vi "Gear Controller.vi"(8 "error in":errorcluster) -> ()   [LabVIEW 2015]
doc: "This VI executes continuously carrying out the current operation and responding to updates or new operations. It will often contain the timing or control code that is difficult to place directly in TeleOp. This VI generally opens all sensors and motors and isolates the rest of the robot code from knowing how the operations are carried out."
uses:
  Gear.ctl
  <vilib>/Rock Robotics/WPI/Solenoid/WPI_SolenoidValue.ctl
  Gear Setpoints.ctl
  Gear Operations.ctl
  <vilib>/Rock Robotics/WPI/Solenoid/WPI_SolenoidChannel.ctl
  Framework/Robot Global Data.vi
  <vilib>/Rock Robotics/WPI/Solenoid/WPI_SolenoidOpenSingle.vi
  <vilib>/Rock Robotics/WPI/Solenoid/WPI_SolenoidSetEnum.vi
panel:
  out "error IO":errorcluster
  in  "Apply Change":bool
  in  "Solenoid 6 (PTO de-active)":T1
  in  "Solenoid 5 (PTO Active)":T1
  in  "Solenoid 4 (Holdball)":T1
  in  "Solenoid 3 (Shootball)":T1
  in  "Solenoid 2 (Gearbox High)":T1
  in  "Solenoid 1 (Gearbox Low)":T1
  out "Gear":T2
  out "Current\nCmd":string
  # "Tip: It may be helpful to observe inputs and sensor values.\nYou may also want to display tuning or debugging controls."
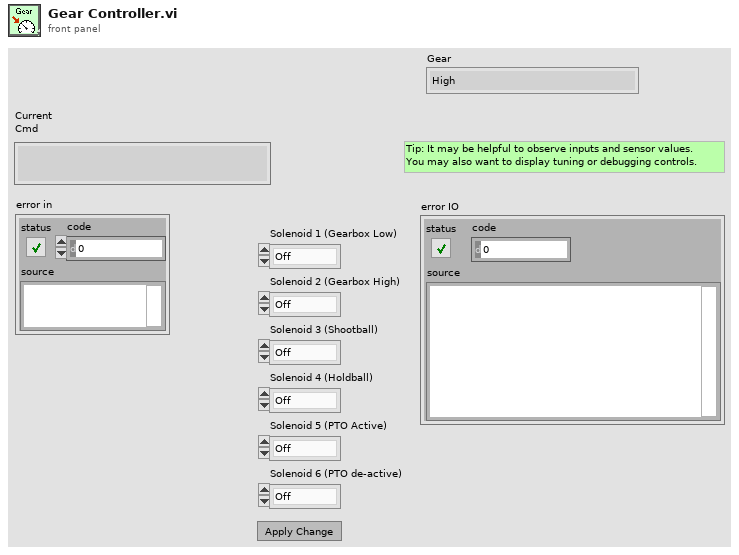
[diagram p1: front panel]
types:
  T1 = typedef "WPI_SolenoidValue.ctl" = enum16{"Off", "On", "Forward", "Reverse"}
  T2 = typedef "Gear.ctl" = enum16{"High", "Low"}
  T3 = typedef "Robot Type Def.ctl" = enum16{"Disabled", "Ghost", "Casper", "Lofty", "Board"}
  T4 = typedef "WPI_SolenoidChannel.ctl" = enum8{"Solenoid 0", "Solenoid 1", "Solenoid 2", "Solenoid 3", "Solenoid 4", "Solenoid 5", "Solenoid 6", "Solenoid 7", "Invalid"}
  T5 = typedef "Gear Setpoints.ctl" = cluster{"Operation":T6, "Setpoint":dbl, "Duration":dbl, "Gear":T2}
  T6 = typedef "Gear Operations.ctl" = enum16{"Reserve", "Read Current", "Immediate", "Change Gear"}
  T7 = typedef "WPI_CompressorDevRef.ctl" = cluster{"DevStatus":errorcluster, "Pneumatics Control Module":u8}
  T8 = typedef "WPI_SolenoidDevRef.ctl" = cluster{"DevStatus":errorcluster, "Pneumatics Control Module":u8, "Forward Solenoid Channel":T4, "Reverse Solenoid Channel":T4}
  T9 = typedef "Command Status Info.ctl" = cluster{"Name":string, "Status":T10, "notifier out":T11}
  T10 = typedef "Completion Status.ctl" = enum16{"Successful", "Aborted", "Incomplete"}
  T11 = typedef "Completion Notifier.ctl" = refnum<notifier>
  T12 = cluster{"Default Command":T5, "Command Timing":cluster{"Start Time (ms)":u32, "Iterations":i32}, "Command Arguments":cluster{"Command Info":T9, "Description":string, "Default Command":T5, "notifier out":refnum<notifier>, "Subsystem Name":string}}
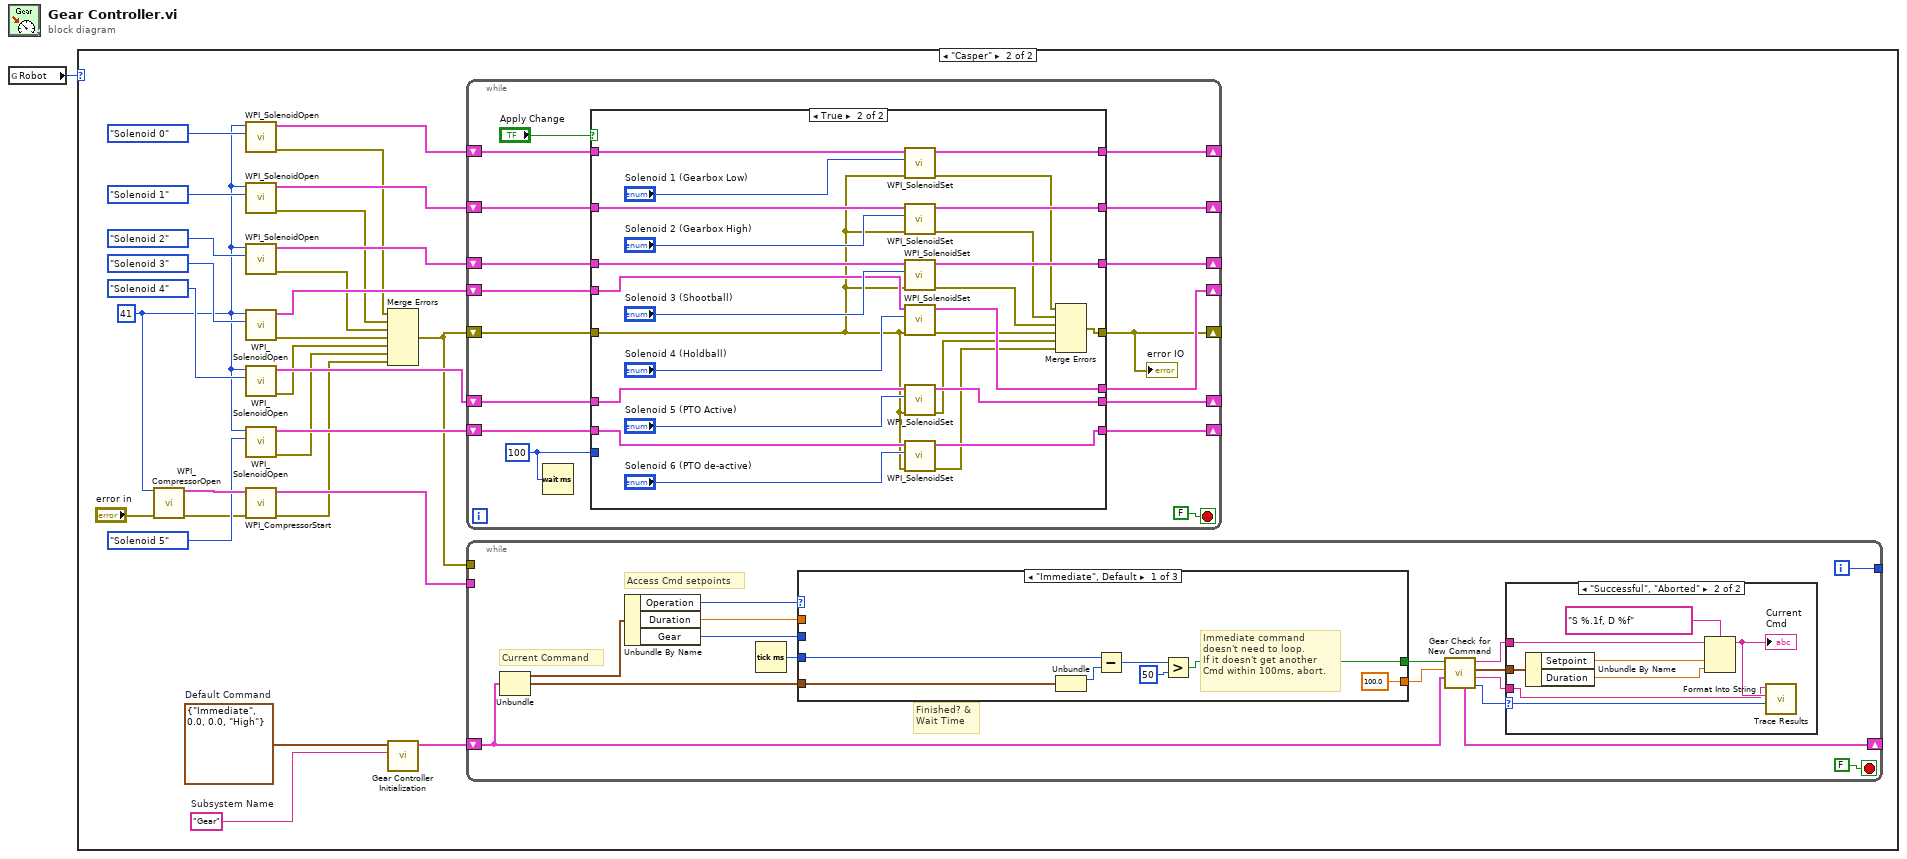
[diagram p0: block diagram]
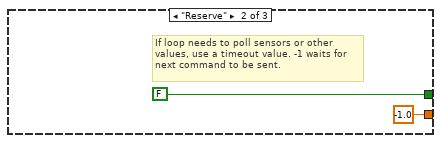
[diagram p5: hidden frame]
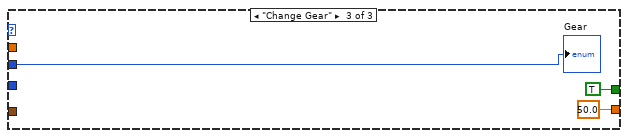
[diagram p6: hidden frame]
diagram:
  n1 = global read "Robot Global Data.vi" "Robot"() -> (w1:T3)
  n2 = case shown="\"Casper\"" w1 {
    frame "Disabled", Default {
    }
    frame "Casper" {
      w17 = u8 41 ("Pneumatics Control Module (0)")
      w27 = T5 {"Operation"=enum."Immediate", "Setpoint"=0.0, "Duration"=0.0, "Gear"=enum."High"}  # Default Command
      w28 = "Gear"  # Subsystem Name
      n3 = call <vilib>:"WPI_CompressorOpen.vi"("Pneumatics Control Module (0)"=w17, "error in (no error)"="error in") -> ("CompressorDevRef"=w26:T7, "error out"=w9:errorcluster)  [unwired: 12 in]
      n4 = call-poly <vilib>:"WPI_SolenoidOpen.vi"("Solenoid Channel"=WPI_SolenoidChannel."Solenoid 0", "Pneumatics Control Module (0)"=w17) -> ("error out"=w2:errorcluster, "SolenoidDevRef"=w23:T8)  [unwired: 8 in]
      n5 = call-poly <vilib>:"WPI_SolenoidOpen.vi"("Solenoid Channel"=WPI_SolenoidChannel."Solenoid 1", "Pneumatics Control Module (0)"=w17) -> ("error out"=w8:errorcluster, "SolenoidDevRef"=w12:T8)  [unwired: 8 in]
      n6 = call-poly <vilib>:"WPI_SolenoidOpen.vi"("Solenoid Channel"=WPI_SolenoidChannel."Solenoid 2", "Pneumatics Control Module (0)"=w17) -> ("error out"=w7:errorcluster, "SolenoidDevRef"=w13:T8)  [unwired: 8 in]
      n7 = call-poly <vilib>:"WPI_SolenoidOpen.vi"("Solenoid Channel"=WPI_SolenoidChannel."Solenoid 3", "Pneumatics Control Module (0)"=w17) -> ("error out"=w6:errorcluster, "SolenoidDevRef"=w14:T8)  [unwired: 8 in]
      n8 = call-poly <vilib>:"WPI_SolenoidOpen.vi"("Solenoid Channel"=WPI_SolenoidChannel."Solenoid 4", "Pneumatics Control Module (0)"=w17) -> ("error out"=w5:errorcluster, "SolenoidDevRef"=w15:T8)  [unwired: 8 in]
      n9 = call-poly <vilib>:"WPI_SolenoidOpen.vi"("Solenoid Channel"=WPI_SolenoidChannel."Solenoid 5", "Pneumatics Control Module (0)"=w17) -> ("error out"=w4:errorcluster, "SolenoidDevRef"=w16:T8)  [unwired: 8 in]
      n10 = call <vilib>:"WPI_CompressorStart.vi"("error in (no error)"=w9, "CompressorDevRef"=w26) -> ("error out"=w3:errorcluster, "CompressorDevRef"=w25:T7)  [unwired: 8 in]
      n11 = Merge Errors(w2, w8, w7, w6, w5, w4, w3) -> (w11:errorcluster)
      n12 = call "Gear Controller Initialization.vi"("Subsystem Name"=w28, "Default Command"=w27) -> ("Command Info"=w29:T12)  [unwired: 9 in]
      n13 = while {
        shift-right: [w45] -> _
        shift-left: w23 -> [w46]
        shift-right: [w39] -> _
        shift-left: w16 -> [w40]
        shift-right: [w38] -> _
        shift-left: w15 -> [w41]
        shift-right: [w37] -> _
        shift-left: w14 -> [w42]
        shift-right: [w36] -> _
        shift-left: w13 -> [w43]
        shift-right: [w35] -> _
        shift-left: w12 -> [w44]
        shift-right: [w32] -> _
        shift-left: w11 -> [w31]
        stop <- FALSE stop-if-true
        w30 = u32 100 ("milliseconds to wait")
        n14 = Wait (ms)(milliseconds to wait=w30) -> ()  [unwired: 1 out]
        n15 = case shown="True" "Apply Change" {
          tunnel: w46 -> [w49 w79]
          tunnel: [w49 w78] -> w45
          tunnel: w44 -> [w50 w75]
          tunnel: w43 -> [w51 w74]
          tunnel: w42 -> [w52 w72]
          tunnel: w41 -> [w53 w69]
          tunnel: w40 -> [w48 w68]
          tunnel: [w48 w66] -> w39
          tunnel: [w53 w65] -> w38
          tunnel: [w52 w64] -> w37
          tunnel: [w51 w63] -> w36
          tunnel: [w50 w62] -> w35
          tunnel: w30 -> [_ _]
          tunnel: [w47 w61] -> w32
          tunnel: w31 -> [w47 w54]
          frame False {
          }
          frame True {
            n16 = call-poly <vilib>:"WPI_SolenoidSet.vi"("error in (no error)"=w54, "Value"="Solenoid 1 (Gearbox Low)", "SolenoidDevRef"=w79) -> ("error out"=w60:errorcluster, "SolenoidDevRef"=w78:T8)  [unwired: 7 in]
            n17 = call-poly <vilib>:"WPI_SolenoidSet.vi"("error in (no error)"=w54, "Value"="Solenoid 2 (Gearbox High)", "SolenoidDevRef"=w75) -> ("error out"=w59:errorcluster, "SolenoidDevRef"=w62:T8)  [unwired: 7 in]
            n18 = call-poly <vilib>:"WPI_SolenoidSet.vi"("error in (no error)"=w54, "Value"="Solenoid 3 (Shootball)", "SolenoidDevRef"=w74) -> ("error out"=w58:errorcluster, "SolenoidDevRef"=w63:T8)  [unwired: 7 in]
            n19 = call-poly <vilib>:"WPI_SolenoidSet.vi"("error in (no error)"=w54, "Value"="Solenoid 4 (Holdball)", "SolenoidDevRef"=w72) -> ("error out"=w57:errorcluster, "SolenoidDevRef"=w64:T8)  [unwired: 7 in]
            n20 = call-poly <vilib>:"WPI_SolenoidSet.vi"("error in (no error)"=w54, "Value"="Solenoid 5 (PTO Active)", "SolenoidDevRef"=w69) -> ("error out"=w56:errorcluster, "SolenoidDevRef"=w65:T8)  [unwired: 7 in]
            n21 = call-poly <vilib>:"WPI_SolenoidSet.vi"("error in (no error)"=w54, "Value"="Solenoid 6 (PTO de-active)", "SolenoidDevRef"=w68) -> ("error out"=w55:errorcluster, "SolenoidDevRef"=w66:T8)  [unwired: 7 in]
            n22 = Merge Errors(w60, w59, w58, w57, w56, w55) -> (w61:errorcluster)
          }
        }
        "error IO" <- w32
      }
      n23 = while {
        shift-right: [w86] -> _
        shift-left: w29 -> [w87]
        tunnel: [w94] -> _
        tunnel: w25 -> [_]
        tunnel: w11 -> [_]
        i -> [w94]
        stop <- FALSE stop-if-true
        # "Current Command"
        # "Access Cmd setpoints"
        # "Finished? &\nWait Time"
        n24 = Unbundle(w87) -> ("Default Command"=w93:T5, "Command Timing"=w89:cluster{"Start Time (ms)":u32, "Iterations":i32})  [unwired: 1 out]
        n25 = Unbundle By Name(w93) -> ("Operation"=w92:T6, "Duration"=w91:dbl, "Gear"=w88:T2)
        n26 = Tick Count (ms)() -> (millisecond timer value=w90:u32)
        n27 = case shown="\"Immediate\", Default" w92 {
          tunnel: [100.0 -1.0 50.0] -> w84
          tunnel: [w104 FALSE ("ignore previous (F)") TRUE ("ignore previous (F)")] -> w85
          tunnel: w89 -> [w106 _ _]
          tunnel: w91 -> [_ _ _]
          tunnel: w90 -> [w105 _ _]
          tunnel: w88 -> [_ _ w115]
          frame "Immediate", Default {
            # "Immediate command\ndoesn't need to loop.\nIf it doesn't get another\nCmd within 100ms, abort."
            n28 = Unbundle(w106) -> ("Start Time (ms)"=w109:u32)  [unwired: 1 out]
            n29 = Subtract(x=w105, y=w109) -> (x-y=w108:u32)
            n30 = Greater?(x=w108, y=u8 50 ("Left Motor")) -> (0:w104:bool)
          }
          frame "Reserve" {
            # "If loop needs to poll sensors or other\nvalues, use a timeout value. -1 waits for\nnext command to be sent."
          }
          frame "Change Gear" {
            "Gear" <- w115
          }
        }
        n31 = call "Gear Check for New Command.vi"("Current Command"=w87, "Wait time (ms)"=w84, "Finished?"=w85) -> ("Completion"=w80:T10, "Subsystem Name"=w81:string, "Current Command"=w82:T5, "Initial Trace String"=w83:string, "NextCommand"=w86:T12)  [unwired: 4 in]
        n32 = case shown="\"Successful\", \"Aborted\"" w80 {
          selector: w80 -> [_ w103]
          tunnel: w83 -> [_ w99]
          tunnel: w82 -> [_ w100]
          tunnel: w81 -> [_ w96]
          frame "Incomplete", Default {
            # "Continuing current command"
          }
          frame "Successful", "Aborted" {
            # "Report and setup for next command"
            n33 = Unbundle By Name(w100) -> ("Setpoint"=w102:dbl, "Duration"=w97:dbl)
            n34 = Format Into String(format string="S %.1f, D %f", initial string=w99, w102, w97) -> (resulting string=w98:string)  [unwired: 1 in, 1 out]
            "Current\nCmd" <- w98
            n35 = call <vilib>:"Trace Results.vi"("Status of previous command"=w103, "Description"=w98, "Subsystem"=w96) -> ()  [unwired: 9 in]
          }
        }
      }
    }
  }
